vi "Recall Column Widths.vi"(7 "error in":errorcluster, 9 "Display State in":T1, 10 "MCListbox Refnum in":refnum<vi>) -> (0 "error out":errorcluster, 3 "MCListbox Refnum out":refnum<vi>)   [LabVIEW 2012, in "ListBox_XControl.xctl"]
doc: "Recall Column widths from properties and apply to facade. Recalls resized state of columns."
uses:
  ListBox_XControl.xctl
  ListBox_State.ctl
  Order Type Def.ctl
  Value Filters.ctl
  <vilib>/Utility/miscctls.llb/LVRowAndColumnTypeDef.ctl
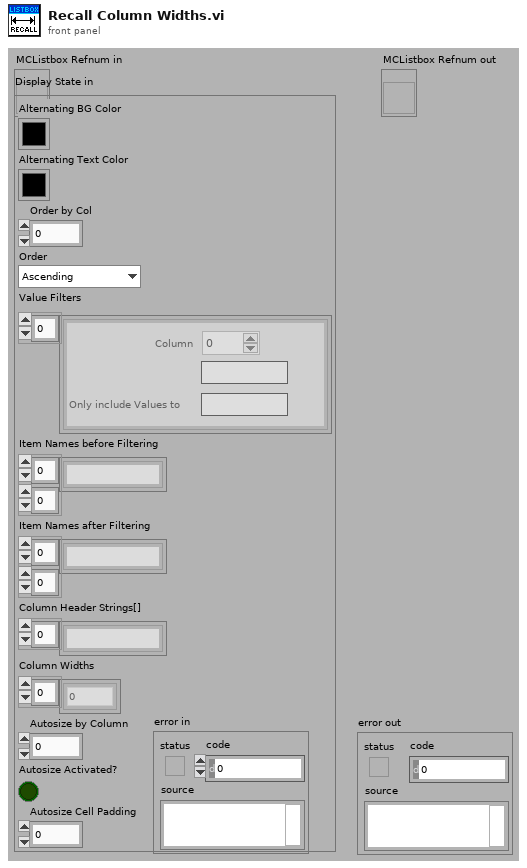
[diagram p1: front panel]
types:
  T1 = typedef "ListBox_XControl.xctl/ListBox_State.ctl" = cluster{"Alternating BG Color":u32, "Alternating Text Color":u32, "Order by Col":i32, "Order":T2, "Value Filters":T3, "Item Names before Filtering":string[][], "Item Names after Filtering":string[][], "Column Header Strings[]":string[], "Column Widths":u32[], "Autosize by Column":i32, "Autosize Activated?":bool, "Autosize Cell Padding":u32}
  T2 = typedef "ListBox_XControl.xctl/Order Type Def.ctl" = enum16{"Ascending", "Descending", "Off"}
  T3 = typedef "ListBox_XControl.xctl/Value Filters.ctl" = cluster{"Column":i32, "Only include Values From":string, "Only include Values to":string}[]
  T4 = typedef "LVRowAndColumnTypeDef.ctl" = cluster{"Row":i32, "Column":i32}
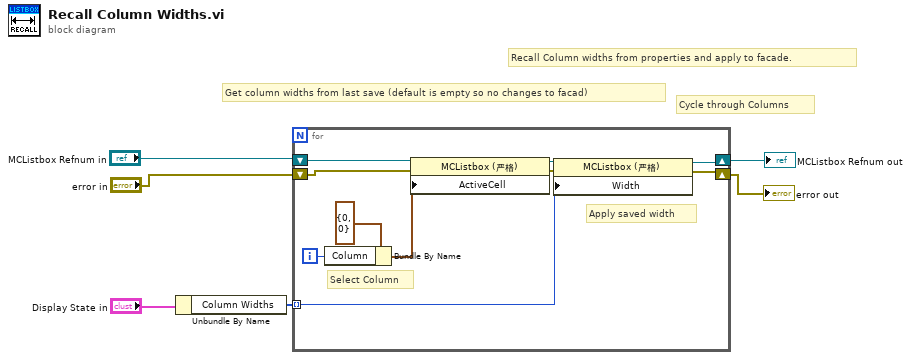
[diagram p0: block diagram]
diagram:
  # "Recall Column widths from properties and apply to facade."
  # "Get column widths from last save (default is empty so no changes to facad)"
  # "Cycle through Columns"
  n1 = Unbundle By Name("Display State in") -> ("Column Widths"=w1:u32[])
  n2 = for {
    shift-right: [w9] -> w5
    shift-left: "error in" -> [w13]
    shift-right: [w8] -> w6
    shift-left: "MCListbox Refnum in" -> [w12]
    tunnel: w1 -> [w7] mode=indexing
    i -> [w16]
    # "Apply saved width"
    # "Select Column"
    n3 = Bundle By Name(cluster=T4 {"Row"=0, "Column"=0} ("Active Cell:Active Cell"), "Column"=w16) -> (w14:T4)
    n4 = property on="Property Node" class="MCListbox (严格)"(reference=w12, error in=w13, "ActiveCell"=w14) -> (reference out=w11:refnum<vi>, error out=w10:errorcluster)
    n5 = property on="Property Node" class="MCListbox (严格)"(reference=w11, error in=w10, "Width"=w7) -> (reference out=w8:refnum<vi>, error out=w9:errorcluster)
  }
  "error out" <- w5
  "MCListbox Refnum out" <- w6
